vi "MotionProfiles_Init.vi"(4 "Wheel_Diameter (in)":dbl=4.0, 6 "MP_Frame_Rate_(ms)":i32=5, 7 "Encoder_CPR_4x":dbl=240.0, 8 "error in (no error)":errorcluster, 9 "CSV File Path":path[](array[path]), 10 "PhoenixMotorControlDevRef":T1={"DeviceStatus"={"status"=FALSE, "code"=0, "source"=""}, "Type"=enum."PWM", "PWM"={"PWM Channel"=enum."Invalid", "DeadBand"={"Name"="", "maxPositivePwm"=0, "minPositivePwm"=0, "centerPwm"=0, "maxNegativePwm"=0, "minNegativePwm"=0, "angularRange"=0}}, "CAN"={"Device Number"=0, "SetOutput VI Ref"=variant(refnum<vi> refnum), "GetOutput VI Ref"=variant(refnum<vi> refnum), "Enable VI Ref"=variant(refnum<vi> refnum), "Disable VI Ref"=variant(refnum<vi> refnum), "Data"=variant}, "Invert"=FALSE, "DIO PWM"={"PWM \"Enable\" Channel"=enum."Invalid", "DIOChannel"=enum."Invalid", "PWM Rate"=0.0}}, 11 "MotionProfiles in":refnum<class "MotionProfiles.lvclass">) -> (0 "error out":errorcluster, 3 "MotionProfiles out":refnum<class "MotionProfiles.lvclass">)   [LabVIEW 2019, in "MotionProfiles.lvclass"]
uses:
  MotionProfiles.lvclass
  <vilib>/Rock Robotics/WPI/MotorControl/WPI_MotorControlDeviceRef.ctl
  <vilib>/Rock Robotics/WPI/MotorControl/WPI_MotorControlType.ctl
  <vilib>/Rock Robotics/SystemInterfaces/DIO/FPGA_DIOPWMChannel.ctl
  <vilib>/Rock Robotics/WPI/PWM/WPI_PWMDeadband.ctl
  <vilib>/Rock Robotics/SystemInterfaces/DIO/FPGA_DIOChannel.ctl
  MotionProfile_InternalStateEnum.ctl
  MotionProfile_TalonSetValueEnum.ctl
  MotionProfile_TrajectoryPoint.ctl
  MotionProfiles.lvclass/MotionProfiles.ctl
  <vilib>/Utility/file.llb/Read Delimited Spreadsheet (DBL).vi
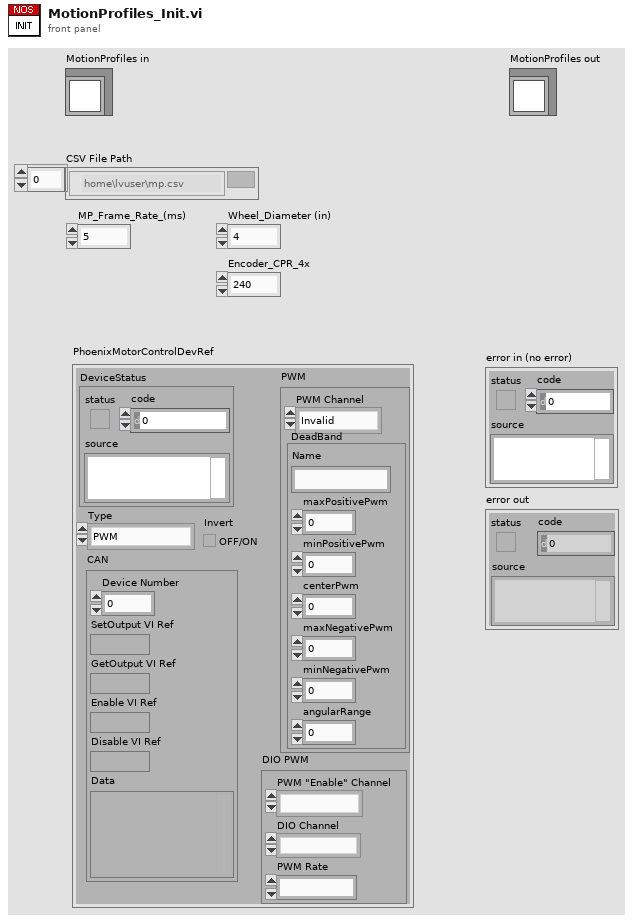
[diagram p1: front panel]
types:
  T1 = typedef "WPI_MotorControlDeviceRef.ctl" = cluster{"DeviceStatus":errorcluster, "Type":T2, "PWM":cluster{"PWM Channel":T3, "DeadBand":T4}, "CAN":cluster{"Device Number":u8, "SetOutput VI Ref":variant, "GetOutput VI Ref":variant, "Enable VI Ref":variant, "Disable VI Ref":variant, "Data":variant}, "Invert":bool, "DIO PWM":cluster{"PWM \"Enable\" Channel":T3, "DIOChannel":T5, "PWM Rate":dbl}}
  T2 = typedef "WPI_MotorControlType.ctl" = enum16{"PWM", "CAN", "DIO PWM"}
  T3 = typedef "FPGA_DIOPWMChannel.ctl" = enum8{"PWM 0", "PWM 1", "PWM 2", "PWM 3", "PWM 4", "PWM 5", "PWM 6", "PWM 7", "PWM 8", "PWM 9", "PWM MXP 0", "PWM MXP 1", "PWM MXP 2", "PWM MXP 3", "PWM MXP 4", "PWM MXP 5", "PWM MXP 6", "PWM MXP 7", "PWM MXP 8", "PWM MXP 9", "Invalid"}
  T4 = typedef "WPI_PWMDeadband.ctl" = cluster{"Name":string, "maxPositivePwm":i32, "minPositivePwm":i32, "centerPwm":i32, "maxNegativePwm":i32, "minNegativePwm":i32, "angularRange":u16}
  T5 = typedef "FPGA_DIOChannel.ctl" = enum8{"DIO 0", "DIO 1", "DIO 2", "DIO 3", "DIO 4", "DIO 5", "DIO 6", "DIO 7", "DIO 8", "DIO 9", "DIO MXP 0", "DIO MXP 1", "DIO MXP 2", "DIO MXP 3", "DIO MXP 4", "DIO MXP 5", "DIO MXP 6", "DIO MXP 7", "DIO MXP 8", "DIO MXP 9", "DIO MXP 10", "DIO MXP 11", "DIO MXP 12", "DIO MXP 13", "DIO MXP 14", "DIO MXP 15", "SPI Port CS1", "SPI Port CS2", "SPI Port CS3", "SPI Port MISO", "SPI Port MOSI", "Invalid"}
  T6 = typedef "MotionProfiles.lvclass/MotionProfile_TrajectoryPoint.ctl" = cluster{"Duration (ms)":u8, "Velocity (u/100ms)":dbl, "Position (units)":dbl, "Profile Slot Select":u8, "Is Last":bool, "Velocity Only":bool, "Zero Position":bool, "Compress Code":u8, "Same Velocity":i32, "Delta Position":i32, "Count":u8, "Invert Motors?":bool}
  T7 = typedef "MotionProfiles.lvclass/MotionProfile_TalonSetValueEnum.ctl" = enum16{"Disable", "Enable", "Hold"}
  T8 = typedef "MotionProfiles.lvclass/MotionProfile_InternalStateEnum.ctl" = enum16{"Nothing", "Send Points to Talon", "Run Profile"}
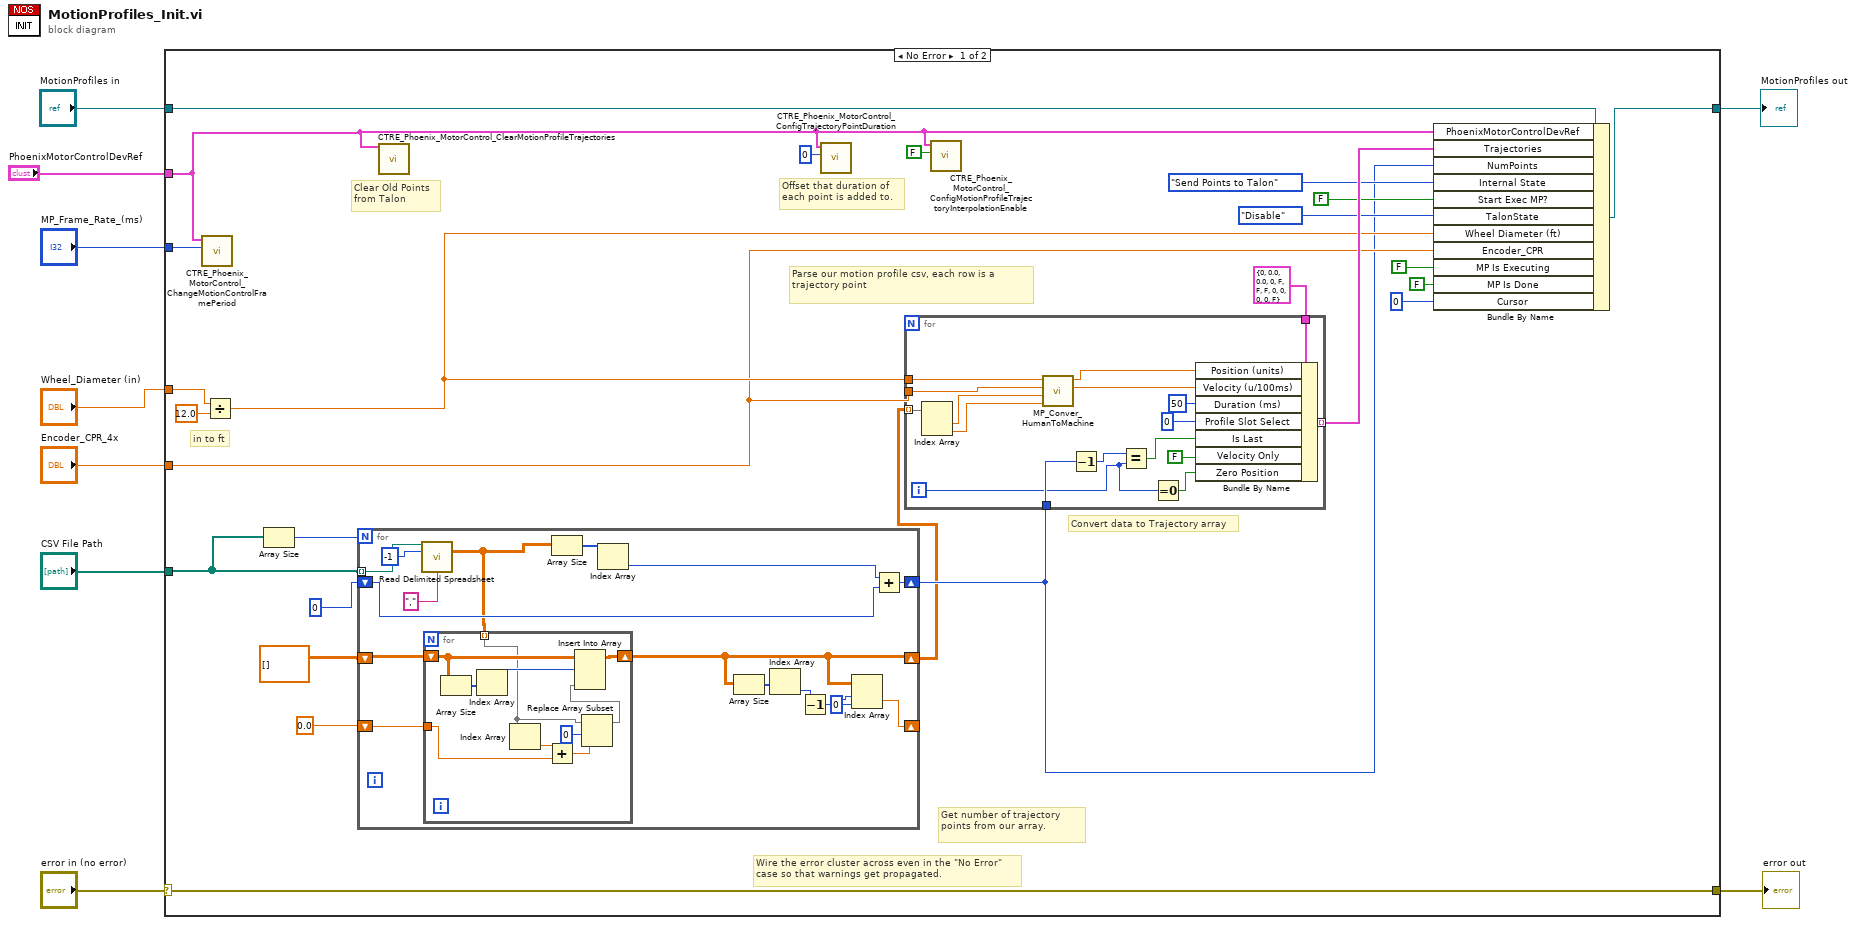
[diagram p0: block diagram]
diagram:
  n1 = case shown="No Error" "error in (no error)" {
    selector: "error in (no error)" -> [w35 w80]
    tunnel: [w35 w80] -> w8
    tunnel: [w34 w79] -> w6
    tunnel: "MotionProfiles in" -> [w27 w79]
    tunnel: "PhoenixMotorControlDevRef" -> [w18 _]
    tunnel: "CSV File Path" -> [w13 _]
    tunnel: "MP_Frame_Rate_(ms)" -> [w26 _]
    tunnel: "Wheel_Diameter (in)" -> [w29 _]
    tunnel: "Encoder_CPR_4x" -> [w19 _]
    frame No Error {
      # "Offset that duration of \neach point is added to."
      # "in to ft"
      # "Clear Old Points\nfrom Talon"
      # "Convert data to Trajectory array"
      # "Get number of trajectory points from our array."
      # "Parse our motion profile csv, each row is a trajectory point"
      # "Wire the error cluster across even in the \"No Error\"\ncase so that warnings get propagated."
      n2 = call <vilib>:"CTRE_Phoenix_MotorControl_ChangeMotionControlFramePeriod.vi"("periodMs"=w26, "PhoenixMotorControlDevRef"=w18) -> ()  [unwired: 8 in, 2 out]
      n3 = Divide(x=w29, y=12.0) -> (x/y=w24:dbl)
      n4 = Array Size(array=w13) -> (size(s)=w14:i32)
      n5 = for {
        N: w14 -> [_]
        tunnel: w13 -> [w50] mode=indexing
        shift-right: [w47] -> w16
        shift-left: 0 -> [w45]
        shift-right: [w41] -> w10
        shift-left: dbl[][] [] ("all rows") -> [w44]
        shift-right: [w39] -> _
        shift-left: 0.0 -> [w36]
        n6 = call-poly <vilib>:"Read Delimited Spreadsheet.vi"("file path (dialog if empty)"=w50, "number of rows (all:-1)"=-1, "delimiter (\\t)"="," ("delimiter (\\t)")) -> ("all rows"=w42:dbl[][])  [unwired: 7 in, 5 out]
        n7 = for {
          tunnel: w42 -> [w55] mode=indexing
          shift-right: [w61] -> w41
          shift-left: w44 -> [w59]
          tunnel: w36 -> [w56]
          n8 = Array Size(array=w59) -> (size(s)=w60:i32[])
          n9 = Index Array(array=w60) -> (element=w58:i32)  [unwired: 1 in]
          n10 = Index Array(array=w55) -> (element=w57:dbl)  [unwired: 1 in]
          n11 = Add(x=w57, y=w56) -> (x+y=w54:dbl)
          n12 = Replace Array Subset(array=w55, new element=w54, index=0) -> (w52:dbl[])
          n13 = Insert Into Array(array=w59, index (row)=w58, new element=w52) -> (w61:dbl[][])  [unwired: 1 in]
        }
        n14 = Array Size(array=w42) -> (size(s)=w48:i32[])
        n15 = Index Array(array=w48) -> (element=w46:i32)  [unwired: 1 in]
        n16 = Array Size(array=w41) -> (size(s)=w43:i32[])
        n17 = Index Array(array=w43) -> (element=w38:i32)  [unwired: 1 in]
        n18 = Decrement(x=w38) -> (x-1=w37:i32)
        n19 = Index Array(array=w41, index (row)=w37, index (col)=0 ("disabled index (col)")) -> (element=w39:dbl)
        n20 = Add(x=w46, y=w45) -> (x+y=w47:i32)
      }
      n21 = call <vilib>:"CTRE_Phoenix_MotorControl_ClearMotionProfileTrajectories.vi"("PhoenixMotorControlDevRef"=w18) -> ()  [unwired: 13 in, 2 out]
      n22 = call <vilib>:"CTRE_Phoenix_MotorControl_ConfigTrajectoryPointDuration.vi"("durationMs"=0, "PhoenixMotorControlDevRef"=w18) -> ()  [unwired: 8 in, 2 out]
      n23 = for {
        tunnel: [w76] -> w33 mode=indexing
        tunnel: w10 -> [w74] mode=indexing
        tunnel: T6 {"Duration (ms)"=0, "Velocity (u/100ms)"=0.0, "Position (units)"=0.0, "Profile Slot Select"=0, "Is Last"=FALSE, "Velocity Only"=FALSE, "Zero Position"=FALSE, "Compress Code"=0, "Same Velocity"=0, "Delta Position"=0, "Count"=0, "Invert Motors?"=FALSE} ("Motion Profile Trajectory Point") -> [w73]
        tunnel: w16 -> [w70]
        tunnel: w24 -> [w69]
        tunnel: w19 -> [w68]
        i -> [w64]
        n24 = Index Array(array=w74) -> (element #1=w67:dbl, element #2=w66:dbl)  [unwired: 2 in]
        n25 = call "MP_Conver_HumanToMachine.vi"("Vel_In (ft/s)"=w66, "Pos_In (ft)"=w67, "CPR"=w68, "Diameter (ft)"=w69) -> ("Vel_Out (u/100ms)"=w65:dbl, "Pos_Out (u)"=w63:dbl)  [unwired: 4 in]
        n26 = Decrement(x=w70) -> (x-1=w71:i32)
        n27 = Equal?(x=w71, y=w64) -> (x = y?=w72:bool)
        n28 = Equal To 0?(x=w64) -> (x = 0?=w77:bool)
        n29 = Bundle By Name(cluster=w73, "Position (units)"=w63, "Velocity (u/100ms)"=w65, "Duration (ms)"=u8 50, "Profile Slot Select"=u8 0, "Is Last"=w72, "Velocity Only"=FALSE, "Zero Position"=w77) -> (w76:T6)
      }
      n30 = call <vilib>:"CTRE_Phoenix_MotorControl_ConfigMotionProfileTrajectoryInterpolationEnable.vi"("enable?"=FALSE, "PhoenixMotorControlDevRef"=w18) -> ()  [unwired: 8 in, 2 out]
      n31 = Bundle By Name(cluster=w27, "PhoenixMotorControlDevRef"=w18, "Trajectories"=w33, "NumPoints"=w16, "Internal State"=MotionProfile_InternalStateEnum."Send Points to Talon", "Start Exec MP?"=FALSE, "TalonState"=MotionProfile_TalonSetValueEnum."Disable" ("TalonSetValue"), "Wheel Diameter (ft)"=w24, "Encoder_CPR"=w19, "MP Is Executing"=FALSE, "MP Is Done"=FALSE, "Cursor"=u32 0) -> (w34:refnum<class "MotionProfiles.lvclass">)
    }
    frame Error {
    }
  }
  "error out" <- w8
  "MotionProfiles out" <- w6
